vi "Reset.vi"(8 "error in (no error)":errorcluster, 10 "restart programs? (false)":bool, 11 "controller in":refnum<k24>) -> (0 "error out":errorcluster, 3 "controller out":refnum<k24>)   [LabVIEW 2020]
uses:
  C:/GEECS/Developers Version/source/Device Drivers/AerotechStage/Sample Vis/Bin/Aerotech.Ensemble.dll
  Sample Vis/Bin/Aerotech.Ensemble.dll
  C:/GEECS/Developers Version/source/Device Drivers/AerotechStage/Sample Vis/Bin/Aerotech.Ensemble.LabVIEW.dll
  Sample Vis/Bin/Aerotech.Ensemble.LabVIEW.dll
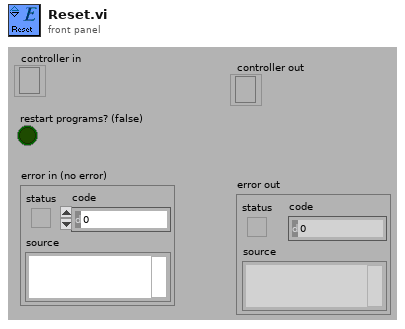
[diagram p1: front panel]
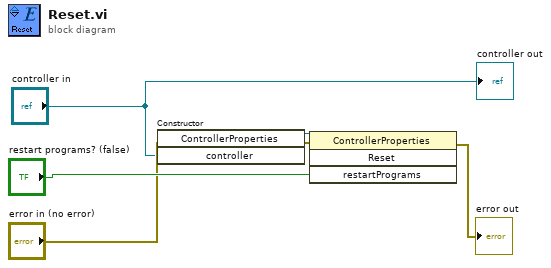
[diagram p0: block diagram]
diagram:
  n1 = constructor class="ControllerProperties"(error in="error in (no error)", "controller"="controller in") -> (reference out=w5:refnum<k24>, error out=w2:errorcluster)  [unwired: 2 in, 2 out]
  n2 = invoke class="ControllerProperties" method="Reset"(reference=w5, error in=w2, "restartPrograms"="restart programs? (false)") -> (error out=→"error out":errorcluster)  [unwired: 1 in, 3 out]
  "controller out" <- "controller in"
